vi "Read Topic Filter.vi"(11 "TopicFilter in":refnum<class "TopicFilter.lvclass">) -> (2 "Topic Filter":string, 3 "TopicFilter out":refnum<class "TopicFilter.lvclass">)   [LabVIEW 2013, in "MQTT Server.lvlib" / "TopicFilter.lvclass"]
uses:
  TopicFilter.lvclass
  TopicFilter.lvclass/TopicFilter.ctl
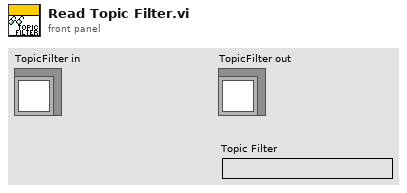
[diagram p1: front panel]
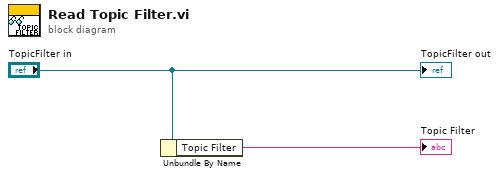
[diagram p0: block diagram]
diagram:
  n1 = Unbundle By Name("TopicFilter in") -> ("Topic Filter"=→"Topic Filter":string)
  "TopicFilter out" <- "TopicFilter in"
